vi "State_Space_Controller.vi"(1 "K5":dbl, 2 "K4":dbl, 3 "K3":dbl, 4 "N":dbl, 5 "K2":dbl, 6 "Reference":dbl, 7 "K1":dbl, 8 "Rads/Sec":dbl, 9 "Rads":dbl, 10 "Meters/Sec":dbl, 11 "Meters":dbl) -> (0 "output":dbl)   [LabVIEW 2016]
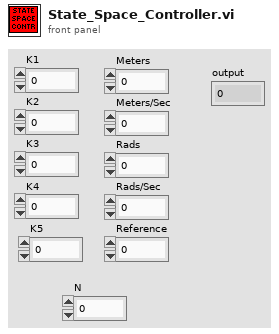
[diagram p1: front panel]
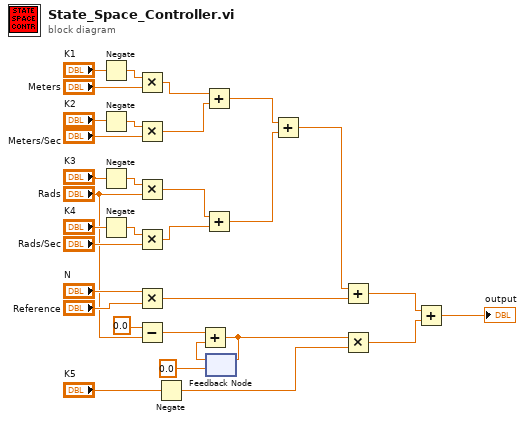
[diagram p0: block diagram]
diagram:
  n1 = Negate(x="K1") -> (-x=w27:dbl)
  n2 = Negate(x="K2") -> (-x=w26:dbl)
  n3 = Negate(x="K3") -> (-x=w24:dbl)
  n4 = Negate(x="K4") -> (-x=w23:dbl)
  n5 = Multiply(x=w27, y="Meters") -> (x*y=w21:dbl)
  n6 = Multiply(x=w26, y="Meters/Sec") -> (x*y=w20:dbl)
  n7 = Multiply(x=w24, y="Rads") -> (x*y=w19:dbl)
  n8 = Multiply(x=w23, y="Rads/Sec") -> (x*y=w18:dbl)
  n9 = Multiply(x="N", y="Reference") -> (x*y=w12:dbl)
  n10 = Subtract(x=0.0, y="Rads") -> (x-y=w9:dbl)
  n11 = Negate(x="K5") -> (-x=w1:dbl)
  n12 = Add(x=w21, y=w20) -> (x+y=w17:dbl)
  n13 = Add(x=w19, y=w18) -> (x+y=w16:dbl)
  n14 = feedback #1(0.0 ("x")) -> (w7:dbl)
  n15 = Add(x=w9, y=w7) -> (x+y=w6:dbl)
  n16 = feedback-in #1(w6) -> ()
  n17 = Add(x=w17, y=w16) -> (x+y=w15:dbl)
  n18 = Add(x=w15, y=w12) -> (x+y=w5:dbl)
  n19 = Multiply(x=w6, y=w1) -> (x*y=w4:dbl)
  n20 = Add(x=w5, y=w4) -> (x+y=→"output":dbl)
